vi "Set XY Graph Value.vi"(9 "XY Graph Data Group In":cluster{"XY Graph Data Group":T1[]} {"XY Graph Data Group"."Y" format="%#_f"; "XY Graph Data Group"."X" format="%#_f"}, 11 "XY Graph Reference In":refnum<vi>) -> ()   [LabVIEW 2024]
uses:
  TypeDef/XY Graph Data.ctl
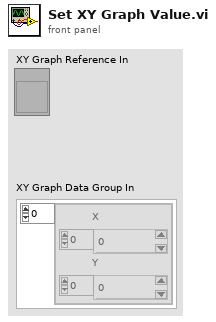
[diagram p1: front panel]
types:
  T1 = typedef "XY Graph Data.ctl" = cluster{"X":dbl[], "Y":dbl[]}
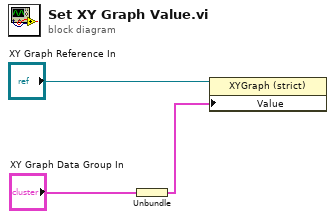
[diagram p0: block diagram]
diagram:
  n1 = Unbundle("XY Graph Data Group In") -> ("XY Graph Data Group"=w1:T1[])
  n2 = property class="XYGraph (strict)"(reference="XY Graph Reference In", "Value"=w1) -> ()  [unwired: 1 in, 2 out]
